vi "manual rf control w diode feedback.vi"() -> ()   [LabVIEW 2018]
uses:
  <vilib>/DAQmx/write.llb/DAQmx Write (Analog DBL 1Chan 1Samp).vi
  <vilib>/DAQmx/read.llb/DAQmx Read (Analog Wfm 1Chan NSamp).vi
  <vilib>/DAQmx/create/channels.llb/DAQmx Create Channel (AO-Voltage-Basic).vi
  <vilib>/DAQmx/create/channels.llb/DAQmx Create Channel (AI-Voltage-Basic).vi
  <vilib>/DAQmx/configure/timing.llb/DAQmx Timing (Sample Clock).vi
  <vilib>/DAQmx/miscellaneous.llb/DAQmx Fill In Error Info.vi
panel:
  out "Waveform Graph":dynamicdata(graph)
  in  "Values to Display":dbl=100.0
  in  "Reigniter 3":dbl step=0.01 format="%.3f"
  in  "Reigniter 2":dbl step=0.1 format="%.3f"
  in  "Reigniter":dbl step=1.0 format="%0.2f"
  in  "Reigniter":tag="Dev1/ao1"
  in  "Main RF":dbl min=0.0 max=0.4 step=0.001 format="%.3f"
  in  "Main RF":tag="Dev1/ao0"
  in  "stop":bool
  in  "Diode":tag="Dev1/ai1"
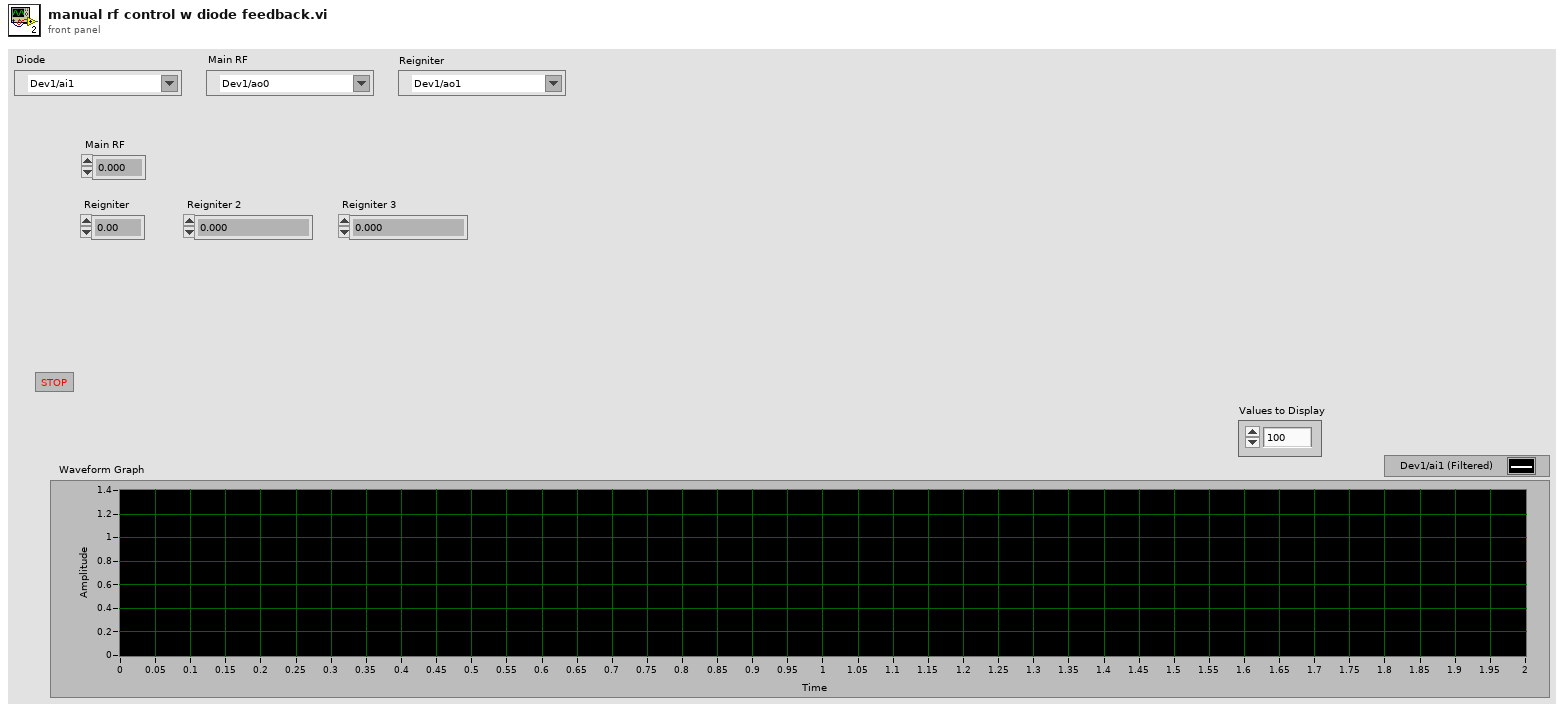
[diagram p1: front panel]
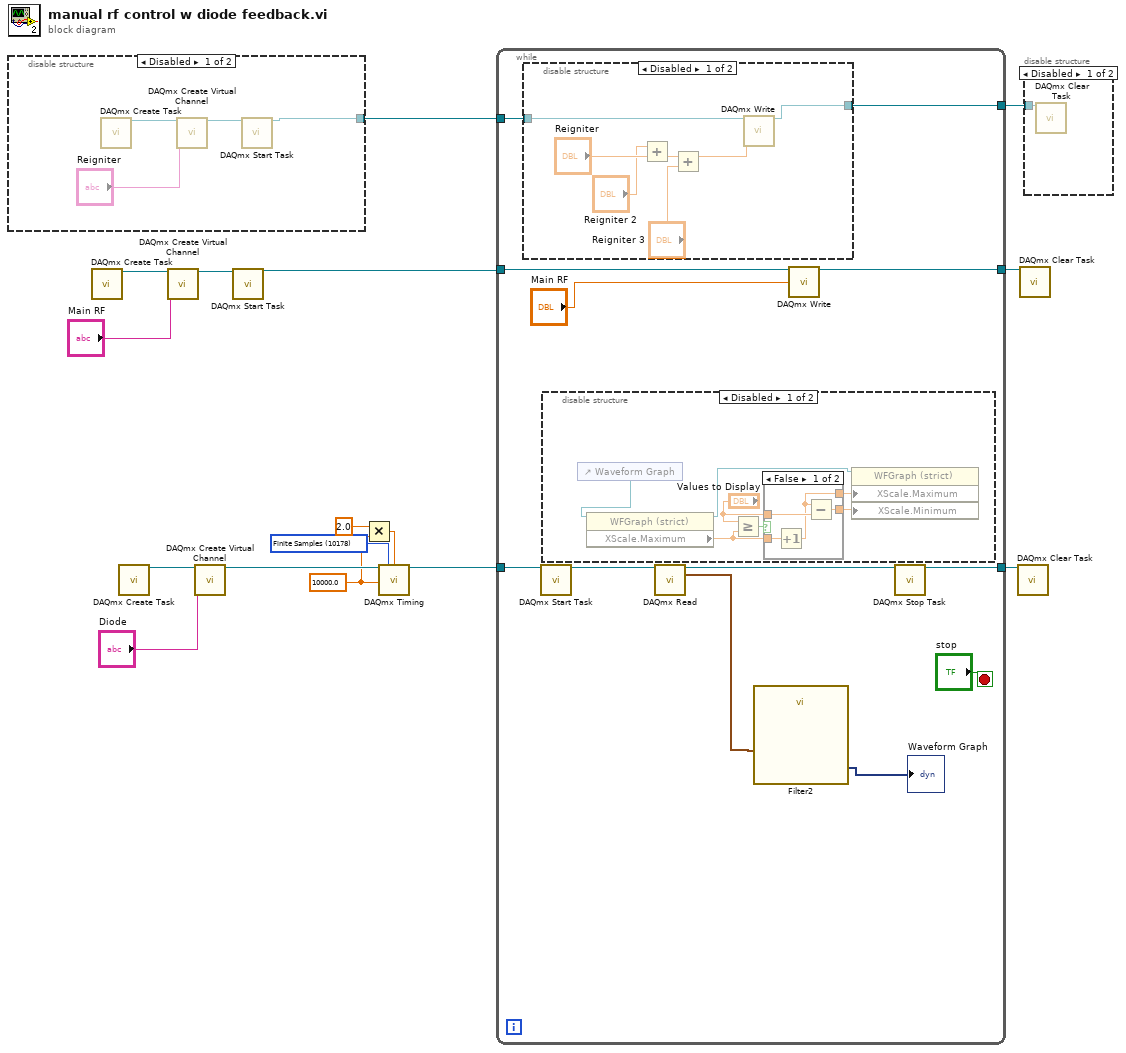
[diagram p0: block diagram]
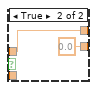
[diagram p5: hidden frame]
diagram:
  w1 = 10178 items=["Finite Samples"=10178, "Continuous Samples"=10123, "Hardware Timed Single Point"=12522] ("sample mode")
  w4 = 10000.0 ("rate")
  n1 = disable-structure shown="Disabled" {
    disable-tunnel: [w17 _] -> w10
    frame Disabled {
      n2 = call <vilib>:"DAQmx Create Task.vi"() -> ("task out"=w20:refnum<k21>)  [unwired: 14 in, 1 out]
      n3 = call-poly <vilib>:"DAQmx Create Virtual Channel.vi"("task in"=w20, "physical channels"="Reigniter") -> ("task out"=w19:refnum<k21>)  [unwired: 12 in, 1 out]
      n4 = call <vilib>:"DAQmx Start Task.vi"("task/channels in"=w19) -> ("task out"=w17:refnum<k21>)  [unwired: 13 in, 1 out]
    }
    frame Enabled {
    }
  }
  n5 = call <vilib>:"DAQmx Create Task.vi"() -> ("task out"=w15:refnum<k21>)  [unwired: 14 in, 1 out]
  n6 = call <vilib>:"DAQmx Create Task.vi"() -> ("task out"=w8:refnum<k21>)  [unwired: 14 in, 1 out]
  n7 = call-poly <vilib>:"DAQmx Create Virtual Channel.vi"("task in"=w15, "physical channels"="Main RF") -> ("task out"=w14:refnum<k21>)  [unwired: 12 in, 1 out]
  n8 = call-poly <vilib>:"DAQmx Create Virtual Channel.vi"("task in"=w8, "physical channels"="Diode") -> ("task out"=w7:refnum<k21>)  [unwired: 12 in, 1 out]
  n9 = call <vilib>:"DAQmx Start Task.vi"("task/channels in"=w14) -> ("task out"=w13:refnum<k21>)  [unwired: 13 in, 1 out]
  n10 = Multiply(x=2.0, y=w4) -> (x*y=w2:dbl)
  n11 = call-poly <vilib>:"DAQmx Timing.vi"("task/channels in"=w7, "sample mode"=w1, "samples per channel"=w2, "rate"=w4) -> ("task out"=w5:refnum<k21>)  [unwired: 10 in, 1 out]
  n12 = while {
    tunnel: w5 -> [w31]
    tunnel: [w23] -> w16
    tunnel: w13 -> [w29]
    tunnel: [w28] -> w12
    tunnel: w10 -> [w26]
    tunnel: [w25] -> w9
    stop <- "stop" stop-if-true
    n13 = disable-structure shown="Disabled" {
      disable-tunnel: w26 -> [w36 _]
      disable-tunnel: [w35 _] -> w25
      frame Disabled {
        n14 = Add(x="Reigniter 2", y="Reigniter") -> (x+y=w38:dbl)
        n15 = Add(x=w38, y="Reigniter 3") -> (x+y=w34:dbl)
        n16 = call-poly <vilib>:"DAQmx Write.vi"("task/channels in"=w36, "data"=w34) -> ("task out"=w35:refnum<k21>)  [unwired: 11 in, 2 out]
      }
      frame Enabled {
      }
    }
    n17 = call <vilib>:"DAQmx Start Task.vi"("task/channels in"=w31) -> ("task out"=w24:refnum<k21>)  [unwired: 13 in, 1 out]
    n18 = disable-structure shown="Disabled" {
      frame Disabled {
        n19 = control-ref of="Waveform Graph"() -> (w40:refnum<vi>)
        n20 = property on="Property Node" class="WFGraph (strict)"(reference=w40) -> (reference out=w41:refnum<vi>, "XScale.Maximum"=w42:dbl)  [unwired: 1 in, 1 out]
        n21 = Greater Or Equal?(x="Values to Display", y=w42) -> (x >= y?=w43:bool)
        n22 = case shown="False" w43 {
          tunnel: "Values to Display" -> [w48 w52]
          tunnel: w42 -> [w50 _]
          tunnel: [w47 w52] -> w45
          tunnel: [w49 0.0] -> w46
          frame False {
            n23 = Increment(x=w50) -> (x+1=w47:dbl)
            n24 = Subtract(x=w47, y=w48) -> (x-y=w49:dbl)
          }
          frame True {
          }
        }
        n25 = property on="Property Node" class="WFGraph (strict)"(reference=w41, "XScale.Maximum"=w45, "XScale.Minimum"=w46) -> ()  [unwired: 1 in, 2 out]
      }
      frame Enabled {
      }
    }
    n26 = call-poly <vilib>:"DAQmx Read.vi"("task/channels in"=w24) -> ("task out"=w30:refnum<k21>, "data"=w22:waveform(dbl))  [unwired: 12 in, 1 out]
    n27 = call "Filter2"("Signal"=w22) -> ("Filtered Signal"=→"Waveform Graph":dynamicdata)  [unwired: 9 in, 1 out]
    n28 = call-poly <vilib>:"DAQmx Write.vi"("task/channels in"=w29, "data"="Main RF") -> ("task out"=w28:refnum<k21>)  [unwired: 11 in, 2 out]
    n29 = call <vilib>:"DAQmx Stop Task.vi"("task/channels in"=w30) -> ("task out"=w23:refnum<k21>)  [unwired: 13 in, 1 out]
  }
  n30 = call <vilib>:"DAQmx Clear Task.vi"("task in"=w16) -> ()  [unwired: 14 in, 1 out]
  n31 = call <vilib>:"DAQmx Clear Task.vi"("task in"=w12) -> ()  [unwired: 14 in, 1 out]
  n32 = disable-structure shown="Disabled" {
    disable-tunnel: w9 -> [w53 _]
    frame Disabled {
      n33 = call <vilib>:"DAQmx Clear Task.vi"("task in"=w53) -> ()  [unwired: 14 in, 1 out]
    }
    frame Enabled {
    }
  }
